vi "Reentrant Config file functional global for GUI elements.vi"(8 "error in":errorcluster, 9 "text to write":string, 10 "file path":path, 11 "Mode":T1=enum."Rewrite file") -> (0 "error out":errorcluster, 1 "text read":string, 2 "file path":path, 3 "Not a Refnum?":bool)   [LabVIEW 2010]
doc: "This RENTRANT .vi handles interactions with the config file (which stores the front panel values) for the various GUI elements (MAIN.vi, SLM Utility, AO tree, etc.)"
uses:
  HHMI - Config file functional global mode enum.ctl
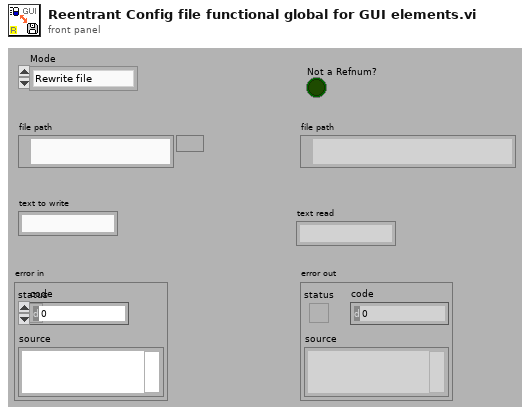
[diagram p1: front panel]
types:
  T1 = typedef "HHMI - Config file functional global mode enum.ctl" = enum16{"Set Filepath", "Read file", "Rewrite file"}
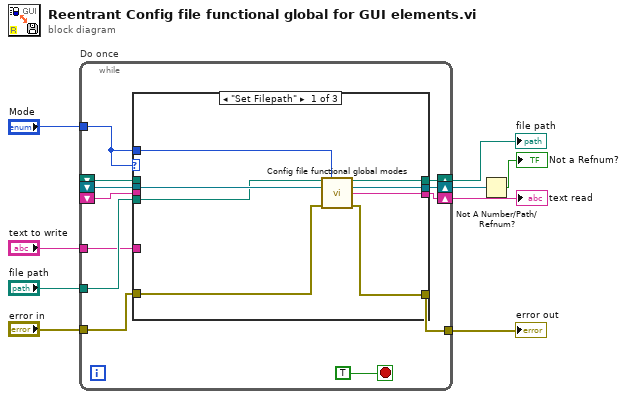
[diagram p0: block diagram]
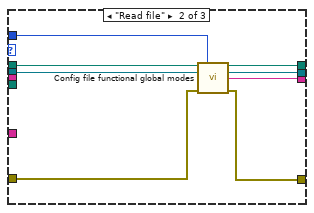
[diagram p2: hidden frame]
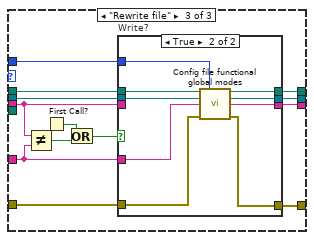
[diagram p3: hidden frame]
diagram:
  n1 = while "Do once" {
    shift-right: [w16] -> w3
    shift-left: _ -> [w15]
    tunnel: "Mode" -> [w11]
    tunnel: "file path" -> [w12]
    shift-right: [w17] -> w2
    shift-left: _ -> [w14]
    tunnel: "error in" -> [w20]
    tunnel: [w19] -> w6
    shift-right: [w18] -> w4
    shift-left: _ -> [w13]
    tunnel: "text to write" -> [w10]
    stop <- TRUE stop-if-true
    n2 = case shown="\"Set Filepath\"" w11 {
      tunnel: w20 -> [w24 w32 w50]
      tunnel: [w26 w34 w49] -> w19
      tunnel: [w25 w33 w48] -> w18
      tunnel: [w27 w35 w47] -> w17
      tunnel: [w28 w36 w46] -> w16
      tunnel: w15 -> [_ w30 w45]
      tunnel: w14 -> [w23 w31 w44]
      tunnel: w11 -> [w29 w37 w43]
      tunnel: w13 -> [_ _ w38]
      tunnel: w12 -> [w22 _ _]
      tunnel: w10 -> [_ _ w39]
      frame "Set Filepath" {
        n3 = call "Config file functional global modes.vi"("File path"=w22, "Mode"=w29, "refnum in"=w23, "error in"=w24) -> ("file path out"=w28:path, "refnum out"=w27:refnum<file>, "text in file"=w25:string, "error out"=w26:errorcluster)  [unwired: 5 in, 3 out]
      }
      frame "Read file" {
        n4 = call "Config file functional global modes.vi"("File path"=w30, "Mode"=w37, "refnum in"=w31, "error in"=w32) -> ("file path out"=w36:path, "refnum out"=w35:refnum<file>, "text in file"=w33:string, "error out"=w34:errorcluster)  [unwired: 4 in, 4 out]
      }
      frame "Rewrite file" {
        n5 = Not Equal?(x=w38, y=w39) -> (x != y?=w42:bool)
        n6 = First Call?() -> (First Call?: T/F=w40:bool)
        n7 = Or(x=w40, y=w42) -> (x .or. y?=w41:bool)
        n8 = case "Write?" shown="True" w41 {
          tunnel: w50 -> [w51 w63]
          tunnel: [w51 w62] -> w49
          tunnel: [w52 w61] -> w48
          tunnel: [w53 w60] -> w47
          tunnel: [w54 w59] -> w46
          tunnel: w45 -> [w54 w58]
          tunnel: w44 -> [w53 w57]
          tunnel: w43 -> [_ w56]
          tunnel: w38 -> [w52 _]
          tunnel: w39 -> [_ w55]
          frame False {
          }
          frame True {
            n9 = call "Config file functional global modes.vi"("File path"=w58, "Mode"=w56, "refnum in"=w57, "text to write"=w55, "error in"=w63) -> ("file path out"=w59:path, "refnum out"=w60:refnum<file>, "text in file"=w61:string, "error out"=w62:errorcluster)  [unwired: 4 in, 3 out]
          }
        }
      }
    }
  }
  "file path" <- w3
  "error out" <- w6
  "text read" <- w4
  n10 = Not A Number/Path/Refnum?(number/path/refnum=w2) -> (NaN/Path/Refnum?=→"Not a Refnum?":bool)
